vi "GVMethode.vi"() -> ()   [LabVIEW 2010]
panel:
  in  "aktuelle Methode":i8
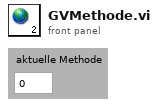
[diagram p1: front panel]
diagram:
